vi "Counter.vi"(10 "Numeric 2":dbl, 11 "State number":dbl) -> (2 "Numeric":dbl)   [LabVIEW 2012]
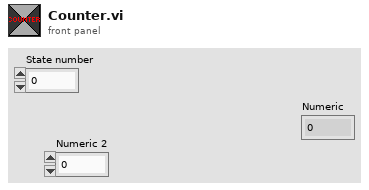
[diagram p1: front panel]
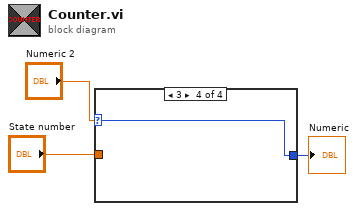
[diagram p0: block diagram]
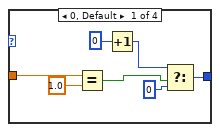
[diagram p2: hidden frame]
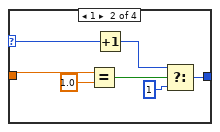
[diagram p3: hidden frame]
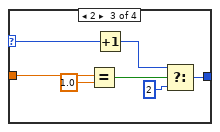
[diagram p4: hidden frame]
diagram:
  n1 = case shown="3" "Numeric 2" {
    selector: "Numeric 2" -> [_ w17 w23 w25]
    tunnel: [w9 w16 w24 w25] -> w2
    tunnel: "State number" -> [w6 w12 w19 _]
    frame 0, Default {
      n2 = Equal?(x=w6, y=1.0) -> (x = y?=w4:bool)
      n3 = Increment(x=0) -> (x+1=w7:i32)
      n4 = Select(t=w7, s=w4, f=0) -> (s? t:f=w9:i32)
    }
    frame 1 {
      n5 = Equal?(x=w12, y=1.0) -> (x = y?=w15:bool)
      n6 = Increment(x=w17) -> (x+1=w14:i32)
      n7 = Select(t=w14, s=w15, f=1) -> (s? t:f=w16:i32)
    }
    frame 2 {
      n8 = Equal?(x=w19, y=1.0) -> (x = y?=w22:bool)
      n9 = Increment(x=w23) -> (x+1=w21:i32)
      n10 = Select(t=w21, s=w22, f=2) -> (s? t:f=w24:i32)
    }
    frame 3 {
    }
  }
  "Numeric" <- w2
